vi "Central Commands.vi"(9 "Value":variant, 10 "Commands":T1, 11 "ref in":refnum<k20>) -> (1 "element":T2, 2 "top enqueue?":bool, 3 "ref out":refnum<k20>)   [LabVIEW 2019]
uses:
  RT Controls/Top Process Commands.ctl
  RT Controls/Top Command Events.ctl
  RT Controls/Main Command Events.ctl
  RT Controls/Main Box Config.ctl
  <vilib>/Utility/error.llb/Error Cluster From Error Code.vi
  <vilib>/rvi/errors/niLvFpgaAdjustHostInterfaceError.vi
  <vilib>/rvi/interface/nirviReadWriteControl/nirviReadWriteControl.xnode
  NiFpgaLv.dll
  <vilib>/rvi/interface/Simulation/niFpgaSimulationCallBeginRW.vi
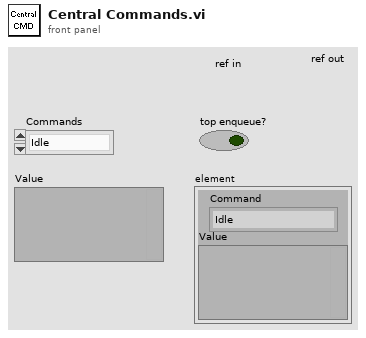
[diagram p1: front panel]
types:
  T1 = typedef "Main Command Events.ctl" = enum16{"Idle", "FullStop", "MainReadConfig", "MainWriteConfig", "OpenUpper", "CloseUpper", "OpenLower", "CloseLower", "SetWatchdogInt", "EnCloudShutDn", "DisCloudShutDn", "SetRainDelay", "EnAutoShutDn", "DisAutoShutDn", "SetRevDelay", "RotToAz", "RotLeft", "RotRight", "RotToHome", "DefineHomePos", "SetHSThres", "SetEncCounts", "SyncClose", "SyncOpen", "SetAZTimLim", "SetAZTol", "AZEncPositive", "AZEncNegative", "RotToCenter"}
  T2 = typedef "Top Process Commands.ctl" = cluster{"Command":T3, "Value":variant}
  T3 = typedef "Top Command Events.ctl" = enum16{"Idle", "FullStop", "ReadConfig", "WriteConfig", "OpenUpper", "CloseUpper", "OpenLower", "CloseLower", "SetWatchdogInt", "EnRainShutDn", "DisRainShutDn", "SetDoorMoveTO", "EnAutoShutDn", "DisAutoShutDn", "SetRevDelay", "SetRainDelay", "SyncClose", "SyncOpen"}
  T4 = typedef "Main Box Config.ctl" = cluster{"WatchdogTim":i32, "DirRevDel":i32, "Coast":dbl, "HSThres":dbl, "EncCounts360":u64, "HomePos":dbl, "EncRefDeg":dbl, "EncRefCounts":u64, "Tol":dbl, "CloudEn":bool, "AutoShutEn":bool, "RainTim":i32, "AZTimeout":i32, "AZEncPol":enum16{"Positive", "Negative"}}
  T5 = cluster{"io.cloud-enable":bool, "io.encoder-negate":bool, "io.encoder-ref":u64, "io.encoder-step":u64, "io.home-pos":fxp<+/-,32,2>, "sm.az-timeout (ms)":u32, "sm.encoder-no-error":u16, "sm.main-pos-hs-thres":fxp<+/-,32,2>, "sm.main-pos-tol":fxp<+/-,32,2>, "sm.cloud-timeout (ms)":u32, "sm.rev-dly (ms)":u32, "io.encoder-center":u64, "sm-main-center-hs-thres":u64, "sm-main-center-tol":u64}
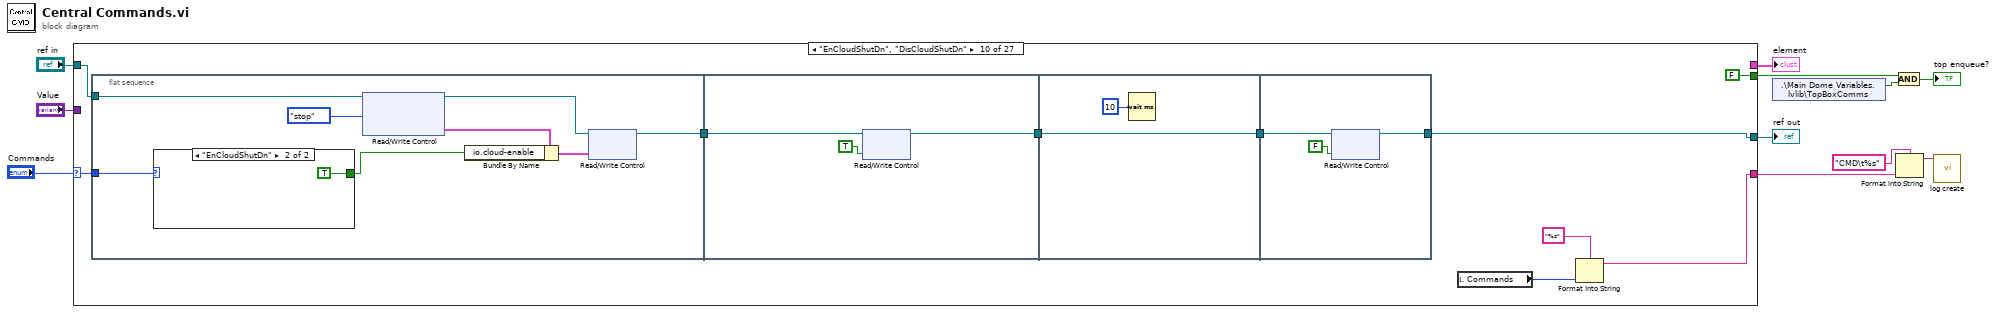
[diagram p0: block diagram]
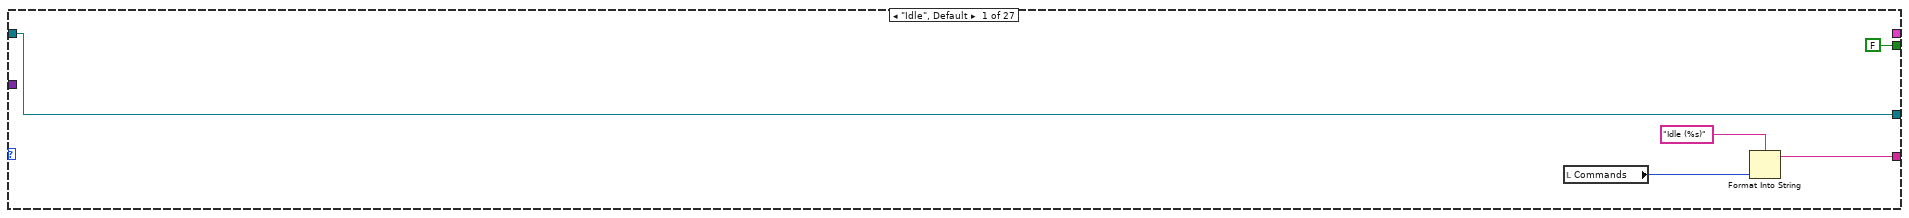
[diagram p2: hidden frame]
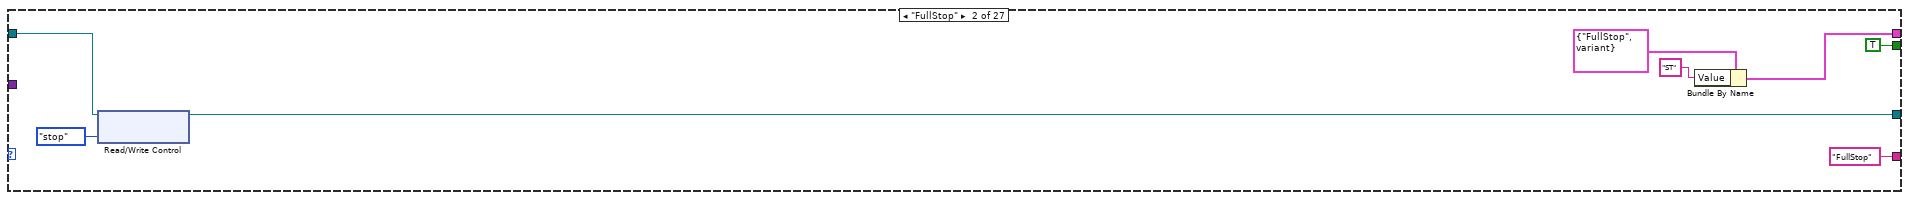
[diagram p3: hidden frame]
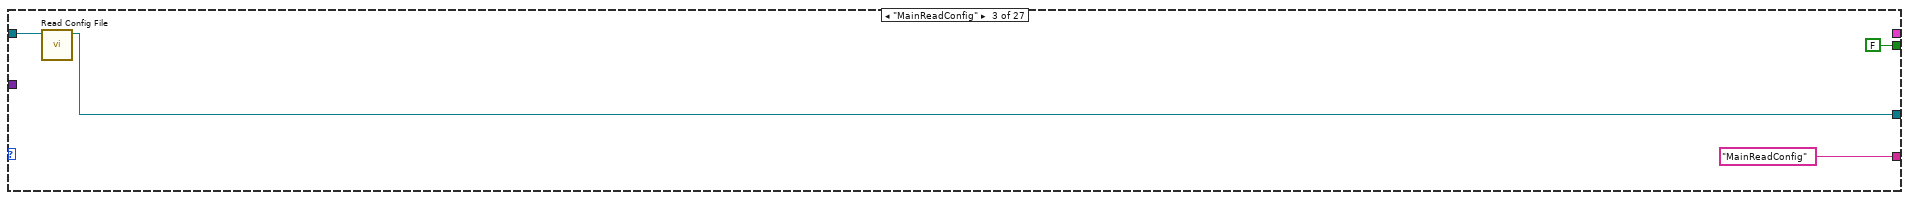
[diagram p4: hidden frame]
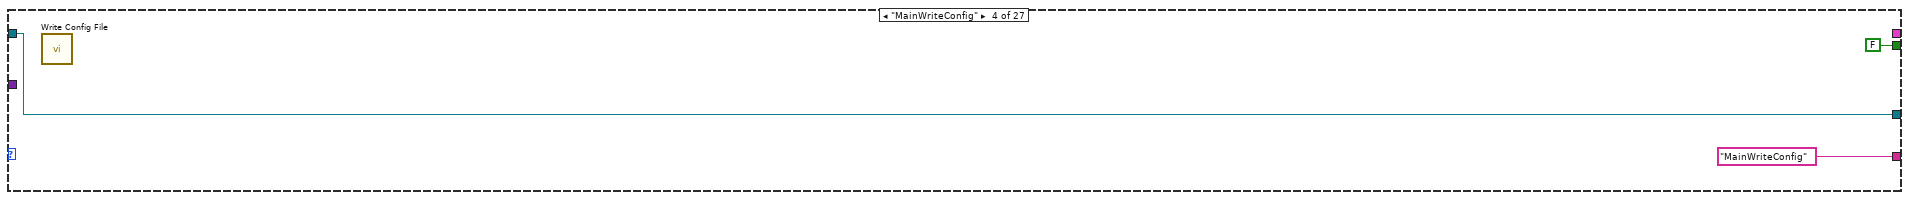
[diagram p5: hidden frame]
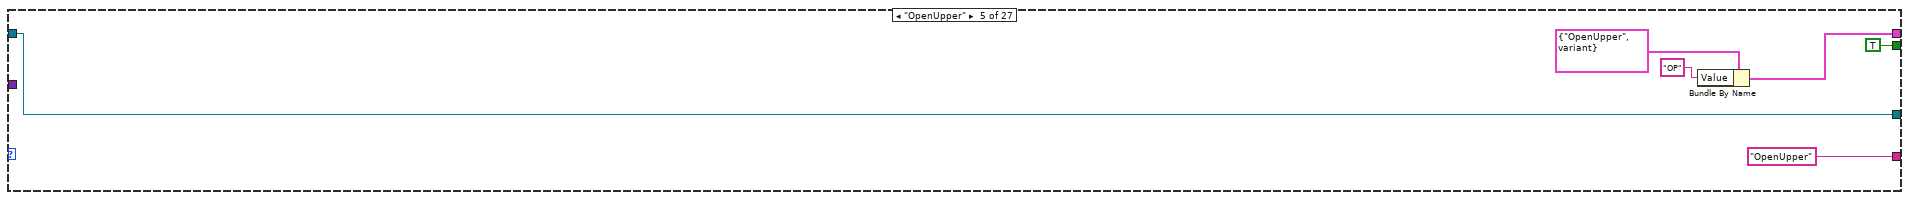
[diagram p6: hidden frame]
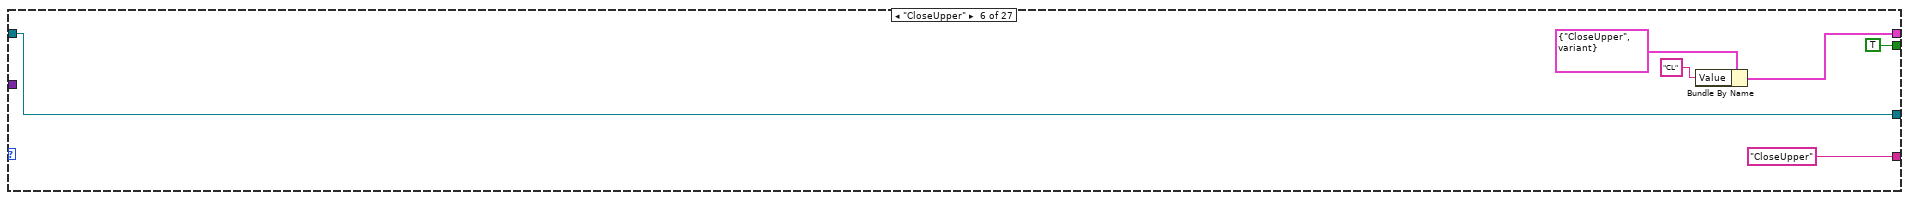
[diagram p7: hidden frame]
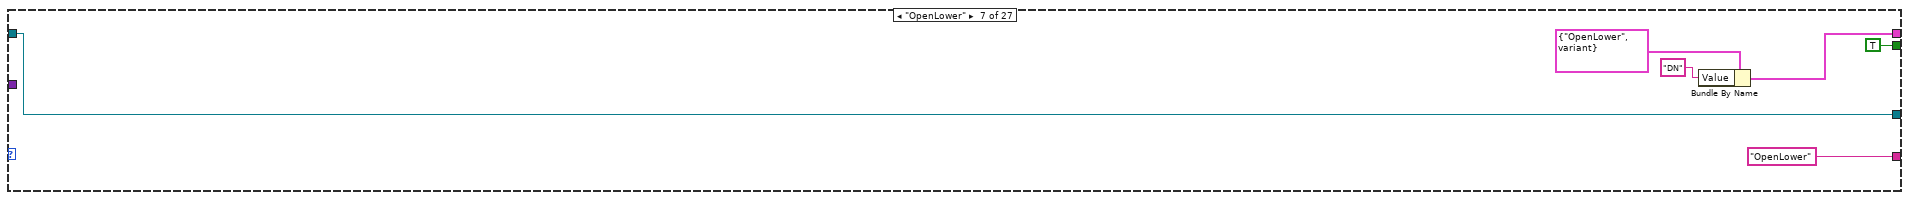
[diagram p8: hidden frame]
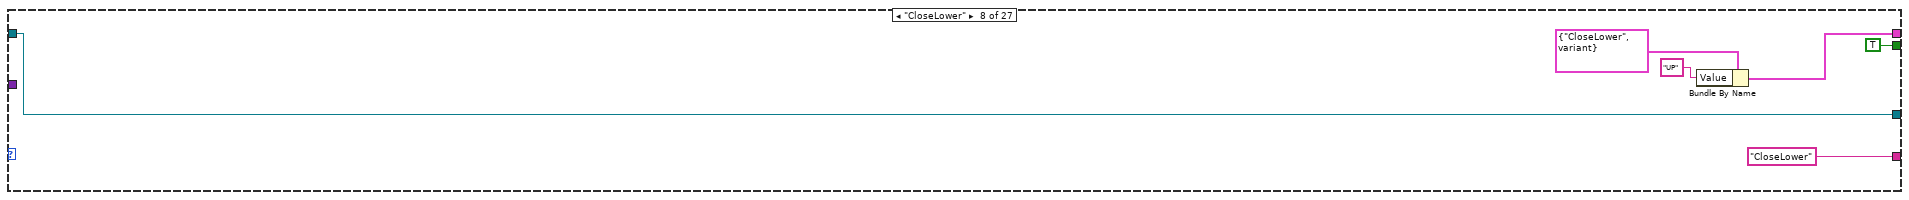
[diagram p9: hidden frame]
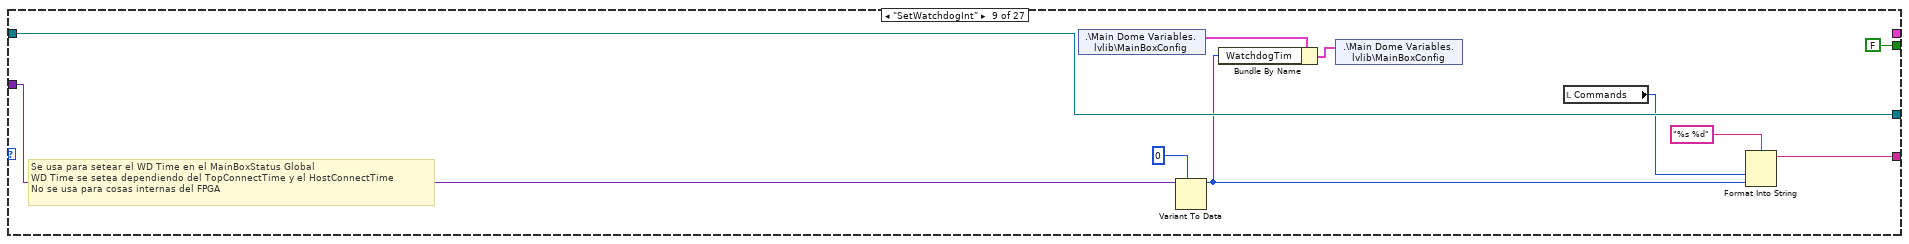
[diagram p10: hidden frame]
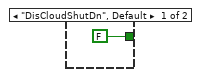
[diagram p11: hidden frame]
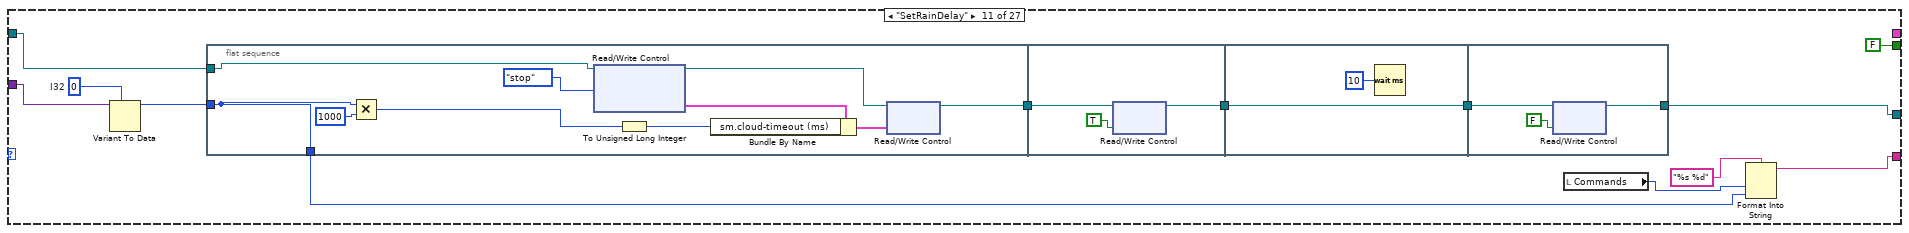
[diagram p12: hidden frame]
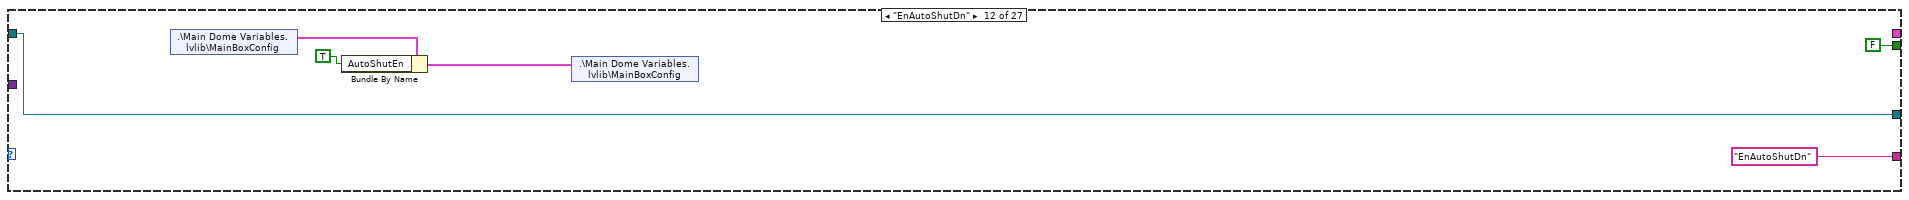
[diagram p13: hidden frame]
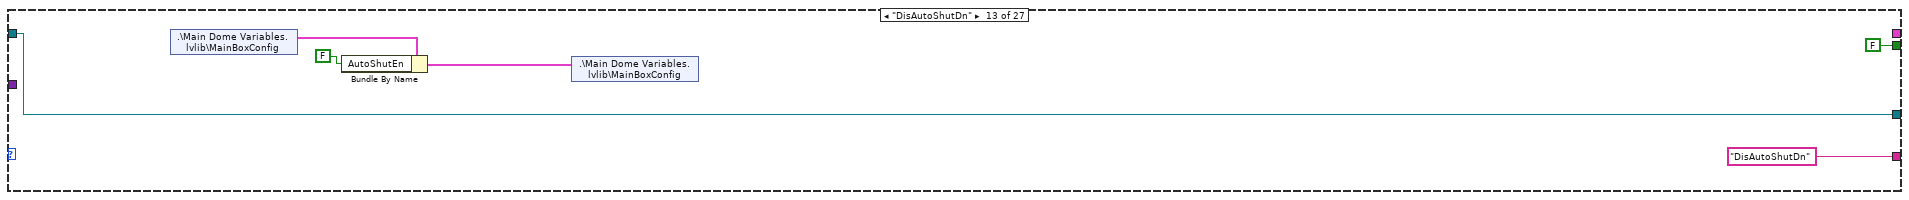
[diagram p14: hidden frame]
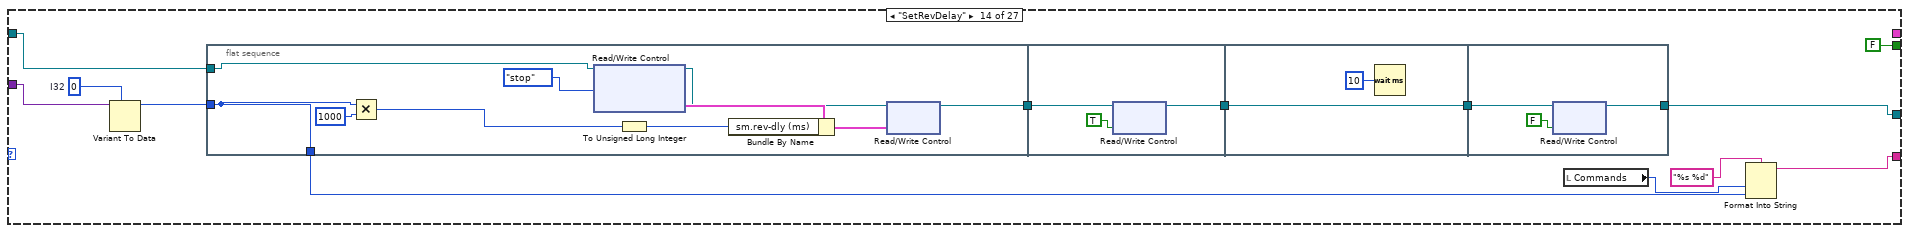
[diagram p15: hidden frame]
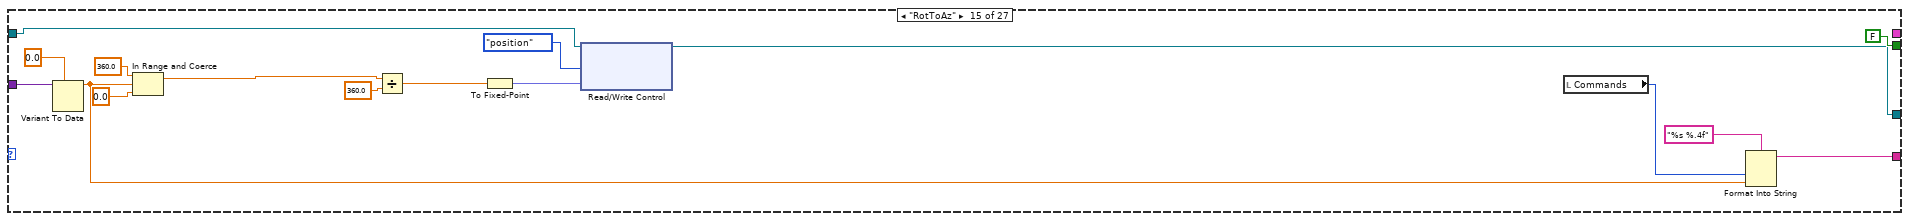
[diagram p16: hidden frame]
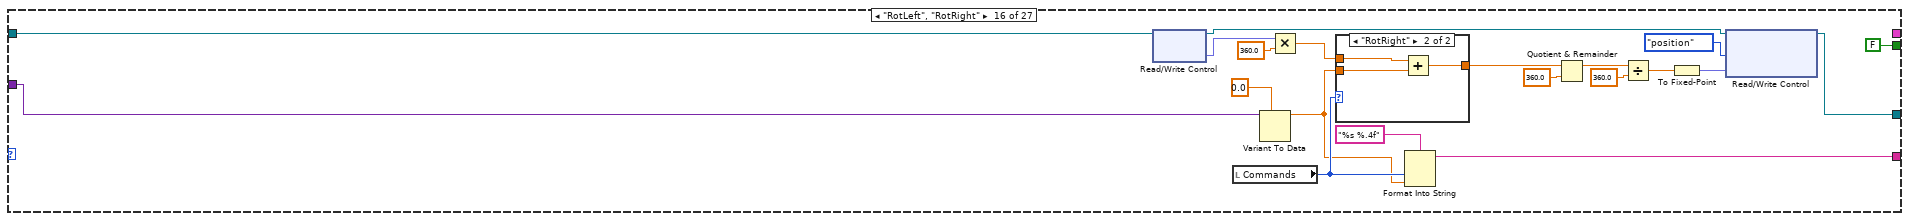
[diagram p17: hidden frame]
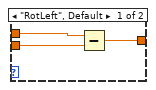
[diagram p18: hidden frame]
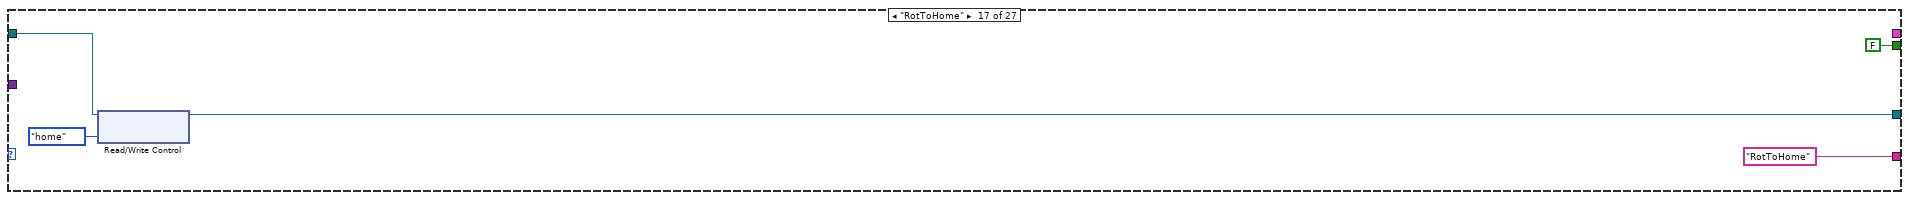
[diagram p19: hidden frame]
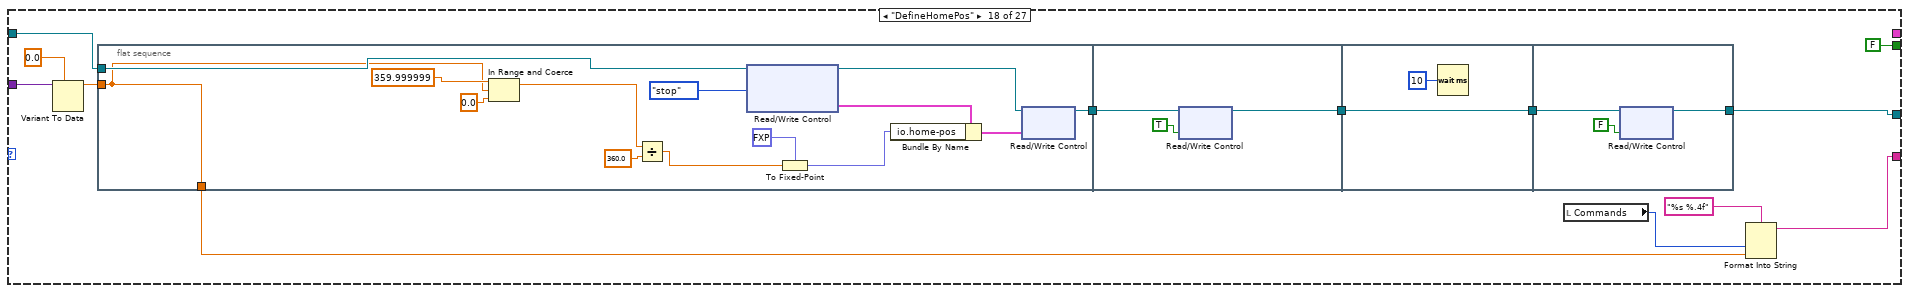
[diagram p20: hidden frame]
diagram:
  n1 = case shown="\"EnCloudShutDn\", \"DisCloudShutDn\"" "Commands" {
    selector: "Commands" -> [_ _ _ _ _ _ _ _ _ w69 _ _ _ _ _ _ _ _ _ _ _ _ _ _ _ _ _]
    tunnel: "Value" -> [_ _ _ _ _ _ _ _ w64 _ w105 _ _ w148 w182 w198 _ w226 w261 w296 _ _ w337 w367 _ _ _]
    tunnel: [FALSE TRUE FALSE FALSE TRUE TRUE TRUE TRUE FALSE FALSE FALSE FALSE FALSE FALSE FALSE FALSE FALSE FALSE FALSE FALSE TRUE TRUE FALSE FALSE FALSE FALSE FALSE] -> w5
    tunnel: [_ w18 _ _ w32 w38 w44 w50 _ _ _ _ _ _ _ _ _ _ _ _ w313 w319 _ _ _ _ _] -> w11
    tunnel: "ref in" -> [w15 w23 w28 w31 w36 w42 w48 w54 w60 w74 w99 w126 w132 w141 w180 w194 w213 w220 w255 w290 w317 w323 w330 w361 w393 w415 w438]
    tunnel: [w15 w22 w27 w31 w36 w42 w48 w54 w60 w70 w98 w126 w132 w143 w173 w197 w212 w219 w254 w289 w317 w323 w329 w360 w392 w414 w437] -> w1
    tunnel: [w12 "FullStop" ("input 1") "MainReadConfig" ("input 1") "MainWriteConfig" ("input 1") "OpenUpper" ("input 1") "CloseUpper" ("input 1") "OpenLower" ("input 1") "CloseLower" ("input 1") w56 w67 w94 "EnAutoShutDn" ("input 1") "DisAutoShutDn" ("input 1") w137 w169 w196 "RotToHome" ("input 1") w215 w250 w285 "SyncClose" ("input 1") "SyncOpen" ("input 1") w325 w356 "AZEncPositive" ("input 1") "AZEncNegative" ("input 1") "RotToCenter" ("input 1")] -> w7
    frame "Idle", Default {
      n2 = local read "Commands"() -> (w13:T1)
      n3 = Format Into String(format string="Idle (%s)", w13) -> (resulting string=w12:string)  [unwired: 2 in, 1 out]
    }
    frame "FullStop" {
      n4 = xnode "Read/Write Control"("FPGA VI Reference In"=w23, "mode request"=enum16{"stop", "home", "position", "center"}."stop") -> ("FPGA VI Reference Out"=w22:refnum<k20>)  [unwired: 1 in, 1 out]
      n5 = Bundle By Name(cluster=T2 {"Command"=enum."FullStop", "Value"=variant} ("element"), "Value"="ST") -> (w18:T2)
    }
    frame "MainReadConfig" {
      n6 = call "Read Config File.vi"("ref in"=w28) -> ("ref out"=w27:refnum<k20>)  [unwired: 10 in]
    }
    frame "MainWriteConfig" {
      n7 = call "Write Config File.vi"() -> ()  [unwired: 12 in]
    }
    frame "OpenUpper" {
      n8 = Bundle By Name(cluster=T2 {"Command"=enum."OpenUpper", "Value"=variant} ("element"), "Value"="OP") -> (w32:T2)
    }
    frame "CloseUpper" {
      n9 = Bundle By Name(cluster=T2 {"Command"=enum."CloseUpper", "Value"=variant} ("element"), "Value"="CL") -> (w38:T2)
    }
    frame "OpenLower" {
      n10 = Bundle By Name(cluster=T2 {"Command"=enum."OpenLower", "Value"=variant} ("element"), "Value"="DN") -> (w44:T2)
    }
    frame "CloseLower" {
      n11 = Bundle By Name(cluster=T2 {"Command"=enum."CloseLower", "Value"=variant} ("element"), "Value"="UP") -> (w50:T2)
    }
    frame "SetWatchdogInt" {
      # "Se usa para setear el WD Time en el MainBoxStatus Global\nWD Time se setea dependiendo del TopConnectTime y el HostConnectTime\nNo se usa para cosas internas del FPGA"
      n12 = shared-variable ".\\Main Dome Variables.lvlib\\MainBoxConfig"() -> (w63:T4)  [unwired: 1 in, 1 out]
      n13 = Variant To Data(type=0 ("number"), Variant=w64) -> (data=w57:i32)  [unwired: 1 in, 1 out]
      n14 = Bundle By Name(cluster=w63, "WatchdogTim"=w57) -> (w62:T4)
      n15 = shared-variable ".\\Main Dome Variables.lvlib\\MainBoxConfig"(w62) -> ()  [unwired: 1 in, 1 out]
      n16 = local read "Commands"() -> (w58:T1)
      n17 = Format Into String(format string="%s %d", w58, w57) -> (resulting string=w56:string)  [unwired: 2 in, 1 out]
    }
    frame "EnCloudShutDn", "DisCloudShutDn" {
      n18 = flat-sequence {
        tunnel: w74 -> [w83]
        tunnel: [w79] -> w73
        tunnel: w69 -> [w78]
        tunnel: w73 -> [w88]
        tunnel: [w86] -> w71
        tunnel: [w89] -> w72
        tunnel: w71 -> [w89]
        tunnel: w72 -> [w92]
        tunnel: [w91] -> w70
        frame #0 {
          n19 = case shown="\"EnCloudShutDn\"" w78 {
            tunnel: [FALSE ("io.cloud-enable") TRUE ("io.cloud-enable")] -> w77
            frame "DisCloudShutDn", Default {
            }
            frame "EnCloudShutDn" {
            }
          }
          n20 = xnode "Read/Write Control"("FPGA VI Reference In"=w83, "mode request"=enum16{"stop", "home", "position", "center"}."stop") -> ("FPGA VI Reference Out"=w81:refnum<k20>, "config"=w82:T5)  [unwired: 1 in, 1 out]
          n21 = Bundle By Name(cluster=w82, "io.cloud-enable"=w77) -> (w80:T5)
          n22 = xnode "Read/Write Control"("FPGA VI Reference In"=w81, "config"=w80) -> ("FPGA VI Reference Out"=w79:refnum<k20>)  [unwired: 1 in, 1 out]
        }
        frame #1 {
          n23 = xnode "Read/Write Control"("FPGA VI Reference In"=w88, "reset"=TRUE) -> ("FPGA VI Reference Out"=w86:refnum<k20>)  [unwired: 1 in, 1 out]
        }
        frame #2 {
          n24 = Wait (ms)(milliseconds to wait=u32 10) -> ()  [unwired: 1 out]
        }
        frame #3 {
          n25 = xnode "Read/Write Control"("FPGA VI Reference In"=w92, "reset"=FALSE) -> ("FPGA VI Reference Out"=w91:refnum<k20>)  [unwired: 1 in, 1 out]
        }
      }
      n26 = local read "Commands"() -> (w66:T1)
      n27 = Format Into String(format string="%s", w66) -> (resulting string=w67:string)  [unwired: 2 in, 1 out]
    }
    frame "SetRainDelay" {
      w106 = 0  # I32
      n28 = Variant To Data(type=w106, Variant=w105) -> (data=w100:i32)  [unwired: 1 in, 1 out]
      n29 = flat-sequence {
        tunnel: w99 -> [w116]
        tunnel: [w112] -> w103
        tunnel: w100 -> [w108]
        tunnel: [w108] -> w95
        tunnel: w103 -> [w119]
        tunnel: [w117] -> w102
        tunnel: [w120] -> w101
        tunnel: w102 -> [w120]
        tunnel: w101 -> [w123]
        tunnel: [w122] -> w98
        frame #0 {
          n30 = Multiply(x=w108, y=1000) -> (x*y=w110:i32)
          n31 = xnode "Read/Write Control"("FPGA VI Reference In"=w116, "mode request"=enum16{"stop", "home", "position", "center"}."stop") -> ("FPGA VI Reference Out"=w114:refnum<k20>, "config"=w115:T5)  [unwired: 1 in, 1 out]
          n32 = To Unsigned Long Integer(number=w110) -> (unsigned 32bit integer=w109:u32)
          n33 = Bundle By Name(cluster=w115, "sm.cloud-timeout (ms)"=w109) -> (w113:T5)
          n34 = xnode "Read/Write Control"("FPGA VI Reference In"=w114, "config"=w113) -> ("FPGA VI Reference Out"=w112:refnum<k20>)  [unwired: 1 in, 1 out]
        }
        frame #1 {
          n35 = xnode "Read/Write Control"("FPGA VI Reference In"=w119, "reset"=TRUE) -> ("FPGA VI Reference Out"=w117:refnum<k20>)  [unwired: 1 in, 1 out]
        }
        frame #2 {
          n36 = Wait (ms)(milliseconds to wait=u32 10) -> ()  [unwired: 1 out]
        }
        frame #3 {
          n37 = xnode "Read/Write Control"("FPGA VI Reference In"=w123, "reset"=FALSE) -> ("FPGA VI Reference Out"=w122:refnum<k20>)  [unwired: 1 in, 1 out]
        }
      }
      n38 = local read "Commands"() -> (w96:T1)
      n39 = Format Into String(format string="%s %d", w96, w95) -> (resulting string=w94:string)  [unwired: 2 in, 1 out]
    }
    frame "EnAutoShutDn" {
      n40 = shared-variable ".\\Main Dome Variables.lvlib\\MainBoxConfig"() -> (w129:T4)  [unwired: 1 in, 1 out]
      n41 = Bundle By Name(cluster=w129, "AutoShutEn"=TRUE ("AllStop")) -> (w128:T4)
      n42 = shared-variable ".\\Main Dome Variables.lvlib\\MainBoxConfig"(w128) -> ()  [unwired: 1 in, 1 out]
    }
    frame "DisAutoShutDn" {
      n43 = shared-variable ".\\Main Dome Variables.lvlib\\MainBoxConfig"() -> (w135:T4)  [unwired: 1 in, 1 out]
      n44 = Bundle By Name(cluster=w135, "AutoShutEn"=FALSE ("AllStop")) -> (w134:T4)
      n45 = shared-variable ".\\Main Dome Variables.lvlib\\MainBoxConfig"(w134) -> ()  [unwired: 1 in, 1 out]
    }
    frame "SetRevDelay" {
      w149 = 0  # I32
      n46 = Variant To Data(type=w149, Variant=w148) -> (data=w142:i32)  [unwired: 1 in, 1 out]
      n47 = flat-sequence {
        tunnel: w141 -> [w159]
        tunnel: [w155] -> w146
        tunnel: w142 -> [w151]
        tunnel: [w151] -> w138
        tunnel: w146 -> [w162]
        tunnel: [w160] -> w145
        tunnel: [w163] -> w144
        tunnel: w145 -> [w163]
        tunnel: w144 -> [w166]
        tunnel: [w165] -> w143
        frame #0 {
          n48 = Multiply(x=w151, y=1000) -> (x*y=w153:i32)
          n49 = xnode "Read/Write Control"("FPGA VI Reference In"=w159, "mode request"=enum16{"stop", "home", "position", "center"}."stop") -> ("FPGA VI Reference Out"=w157:refnum<k20>, "config"=w158:T5)  [unwired: 1 in, 1 out]
          n50 = To Unsigned Long Integer(number=w153) -> (unsigned 32bit integer=w152:u32)
          n51 = Bundle By Name(cluster=w158, "sm.rev-dly (ms)"=w152) -> (w156:T5)
          n52 = xnode "Read/Write Control"("FPGA VI Reference In"=w157, "config"=w156) -> ("FPGA VI Reference Out"=w155:refnum<k20>)  [unwired: 1 in, 1 out]
        }
        frame #1 {
          n53 = xnode "Read/Write Control"("FPGA VI Reference In"=w162, "reset"=TRUE) -> ("FPGA VI Reference Out"=w160:refnum<k20>)  [unwired: 1 in, 1 out]
        }
        frame #2 {
          n54 = Wait (ms)(milliseconds to wait=u32 10) -> ()  [unwired: 1 out]
        }
        frame #3 {
          n55 = xnode "Read/Write Control"("FPGA VI Reference In"=w166, "reset"=FALSE) -> ("FPGA VI Reference Out"=w165:refnum<k20>)  [unwired: 1 in, 1 out]
        }
      }
      n56 = local read "Commands"() -> (w139:T1)
      n57 = Format Into String(format string="%s %d", w139, w138) -> (resulting string=w137:string)  [unwired: 2 in, 1 out]
    }
    frame "RotToAz" {
      n58 = Variant To Data(type=0.0 ("upper limit"), Variant=w182) -> (data=w170:dbl)  [unwired: 1 in, 1 out]
      n59 = In Range and Coerce(upper limit=360.0, x=w170, lower limit=0.0) -> (coerced(x)=w177:dbl)  [unwired: 1 out]
      n60 = Divide(x=w177, y=360.0) -> (x/y=w175:dbl)
      n61 = To Fixed-Point(number=w175) -> (fixed-point=w174:fxp<+/-,32,2>)  [unwired: 1 in]
      n62 = xnode "Read/Write Control"("FPGA VI Reference In"=w180, "mode request"=enum16{"stop", "home", "position", "center"}."position", "az pos req"=w174) -> ("FPGA VI Reference Out"=w173:refnum<k20>)  [unwired: 1 in, 1 out]
      n63 = local read "Commands"() -> (w171:T1)
      n64 = Format Into String(format string="%s %.4f", w171, w170) -> (resulting string=w169:string)  [unwired: 2 in, 1 out]
    }
    frame "RotLeft", "RotRight" {
      n65 = xnode "Read/Write Control"("FPGA VI Reference In"=w194) -> ("FPGA VI Reference Out"=w193:refnum<k20>, "az pos"=w191:fxp<+/-,32,2>)  [unwired: 1 in, 1 out]
      n66 = local read "Commands"() -> (w190:T1)
      n67 = Variant To Data(type=0.0 ("upper limit"), Variant=w198) -> (data=w188:dbl)  [unwired: 1 in, 1 out]
      n68 = Multiply(x=w191, y=360.0 ("upper limit")) -> (x*y=w189:dbl)
      n69 = case shown="\"RotRight\"" w190 {
        tunnel: w189 -> [w205 w209]
        tunnel: w188 -> [w206 w208]
        tunnel: [w204 w207] -> w187
        frame "RotLeft", Default {
          n70 = Subtract(x=w205, y=w206) -> (x-y=w204:dbl)
        }
        frame "RotRight" {
          n71 = Add(x=w209, y=w208) -> (x+y=w207:dbl)
        }
      }
      n72 = Format Into String(format string="%s %.4f", w190, w188) -> (resulting string=w196:string)  [unwired: 2 in, 1 out]
      n73 = Quotient & Remainder(x=w187, y=360.0) -> (x-y*floor(x/y)=w185:dbl)  [unwired: 1 out]
      n74 = Divide(x=w185, y=360.0) -> (x/y=w203:dbl)
      n75 = To Fixed-Point(number=w203) -> (fixed-point=w202:fxp<+/-,32,2>)  [unwired: 1 in]
      n76 = xnode "Read/Write Control"("FPGA VI Reference In"=w193, "mode request"=enum16{"stop", "home", "position", "center"}."position", "az pos req"=w202) -> ("FPGA VI Reference Out"=w197:refnum<k20>)  [unwired: 1 in, 1 out]
    }
    frame "RotToHome" {
      n77 = xnode "Read/Write Control"("FPGA VI Reference In"=w213, "mode request"=enum16{"stop", "home", "position", "center"}."home") -> ("FPGA VI Reference Out"=w212:refnum<k20>)  [unwired: 1 in, 1 out]
    }
    frame "DefineHomePos" {
      n78 = Variant To Data(type=0.0 ("upper limit"), Variant=w226) -> (data=w221:dbl)  [unwired: 1 in, 1 out]
      n79 = flat-sequence {
        tunnel: w220 -> [w241]
        tunnel: [w237] -> w224
        tunnel: w221 -> [w229]
        tunnel: [w229] -> w216
        tunnel: w224 -> [w244]
        tunnel: [w242] -> w223
        tunnel: [w245] -> w222
        tunnel: w223 -> [w245]
        tunnel: w222 -> [w248]
        tunnel: [w247] -> w219
        frame #0 {
          n80 = In Range and Coerce(upper limit=359.999999, x=w229, lower limit=0.0) -> (coerced(x)=w234:dbl)  [unwired: 1 out]
          n81 = Divide(x=w234, y=360.0) -> (x/y=w232:dbl)
          n82 = xnode "Read/Write Control"("FPGA VI Reference In"=w241, "mode request"=enum16{"stop", "home", "position", "center"}."stop") -> ("FPGA VI Reference Out"=w239:refnum<k20>, "config"=w240:T5)  [unwired: 1 in, 1 out]
          n83 = To Fixed-Point(fixed-point type=fxp<+/-,32,2> 0.0 ("az pos req"), number=w232) -> (fixed-point=w230:fxp<+/-,32,2>)
          n84 = Bundle By Name(cluster=w240, "io.home-pos"=w230) -> (w238:T5)
          n85 = xnode "Read/Write Control"("FPGA VI Reference In"=w239, "config"=w238) -> ("FPGA VI Reference Out"=w237:refnum<k20>)  [unwired: 1 in, 1 out]
        }
        frame #1 {
          n86 = xnode "Read/Write Control"("FPGA VI Reference In"=w244, "reset"=TRUE) -> ("FPGA VI Reference Out"=w242:refnum<k20>)  [unwired: 1 in, 1 out]
        }
        frame #2 {
          n87 = Wait (ms)(milliseconds to wait=u32 10) -> ()  [unwired: 1 out]
        }
        frame #3 {
          n88 = xnode "Read/Write Control"("FPGA VI Reference In"=w248, "reset"=FALSE) -> ("FPGA VI Reference Out"=w247:refnum<k20>)  [unwired: 1 in, 1 out]
        }
      }
      n89 = local read "Commands"() -> (w217:T1)
      n90 = Format Into String(format string="%s %.4f", w217, w216) -> (resulting string=w215:string)  [unwired: 2 in, 1 out]
    }
    frame "SetHSThres" {
      n91 = Variant To Data(type=0.0 ("upper limit"), Variant=w261) -> (data=w256:dbl)  [unwired: 1 in, 1 out]
      n92 = flat-sequence {
        tunnel: w255 -> [w276]
        tunnel: [w272] -> w259
        tunnel: w256 -> [w264]
        tunnel: [w264] -> w251
        tunnel: w259 -> [w279]
        tunnel: [w277] -> w258
        tunnel: [w280] -> w257
        tunnel: w258 -> [w280]
        tunnel: w257 -> [w283]
        tunnel: [w282] -> w254
        frame #0 {
          n93 = In Range and Coerce(upper limit=359.999999, x=w264, lower limit=0.0) -> (coerced(x)=w269:dbl)  [unwired: 1 out]
          n94 = Divide(x=w269, y=360.0) -> (x/y=w267:dbl)
          n95 = xnode "Read/Write Control"("FPGA VI Reference In"=w276, "mode request"=enum16{"stop", "home", "position", "center"}."stop") -> ("FPGA VI Reference Out"=w274:refnum<k20>, "config"=w275:T5)  [unwired: 1 in, 1 out]
          n96 = To Fixed-Point(fixed-point type=fxp<+/-,32,2> 0.0 ("az pos req"), number=w267) -> (fixed-point=w265:fxp<+/-,32,2>)
          n97 = Bundle By Name(cluster=w275, "sm.main-pos-hs-thres"=w265) -> (w273:T5)
          n98 = xnode "Read/Write Control"("FPGA VI Reference In"=w274, "config"=w273) -> ("FPGA VI Reference Out"=w272:refnum<k20>)  [unwired: 1 in, 1 out]
        }
        frame #1 {
          n99 = xnode "Read/Write Control"("FPGA VI Reference In"=w279, "reset"=TRUE) -> ("FPGA VI Reference Out"=w277:refnum<k20>)  [unwired: 1 in, 1 out]
        }
        frame #2 {
          n100 = Wait (ms)(milliseconds to wait=u32 10) -> ()  [unwired: 1 out]
        }
        frame #3 {
          n101 = xnode "Read/Write Control"("FPGA VI Reference In"=w283, "reset"=FALSE) -> ("FPGA VI Reference Out"=w282:refnum<k20>)  [unwired: 1 in, 1 out]
        }
      }
      n102 = local read "Commands"() -> (w252:T1)
      n103 = Format Into String(format string="%s %.4f", w252, w251) -> (resulting string=w250:string)  [unwired: 2 in, 1 out]
    }
    frame "SetEncCounts" {
      n104 = Variant To Data(type=u64 0 ("upper limit"), Variant=w296) -> (data=w291:u64)  [unwired: 1 in, 1 out]
      n105 = flat-sequence {
        tunnel: w290 -> [w304]
        tunnel: [w300] -> w294
        tunnel: w291 -> [w299]
        tunnel: [w299] -> w287
        tunnel: w294 -> [w307]
        tunnel: [w305] -> w293
        tunnel: [w308] -> w292
        tunnel: w293 -> [w308]
        tunnel: w292 -> [w311]
        tunnel: [w310] -> w289
        frame #0 {
          n106 = xnode "Read/Write Control"("FPGA VI Reference In"=w304, "mode request"=enum16{"stop", "home", "position", "center"}."stop") -> ("FPGA VI Reference Out"=w302:refnum<k20>, "config"=w303:T5)  [unwired: 1 in, 1 out]
          n107 = Bundle By Name(cluster=w303, "io.encoder-step"=w299) -> (w301:T5)
          n108 = xnode "Read/Write Control"("FPGA VI Reference In"=w302, "config"=w301) -> ("FPGA VI Reference Out"=w300:refnum<k20>)  [unwired: 1 in, 1 out]
        }
        frame #1 {
          n109 = xnode "Read/Write Control"("FPGA VI Reference In"=w307, "reset"=TRUE) -> ("FPGA VI Reference Out"=w305:refnum<k20>)  [unwired: 1 in, 1 out]
        }
        frame #2 {
          n110 = Wait (ms)(milliseconds to wait=u32 10) -> ()  [unwired: 1 out]
        }
        frame #3 {
          n111 = xnode "Read/Write Control"("FPGA VI Reference In"=w311, "reset"=FALSE) -> ("FPGA VI Reference Out"=w310:refnum<k20>)  [unwired: 1 in, 1 out]
        }
      }
      n112 = local read "Commands"() -> (w286:T1)
      n113 = Format Into String(format string="%s %d", w286, w287) -> (resulting string=w285:string)  [unwired: 2 in, 1 out]
    }
    frame "SyncClose" {
      n114 = Bundle By Name(cluster=T2 {"Command"=enum."SyncClose", "Value"=variant} ("element"), "Value"="SC") -> (w313:T2)
    }
    frame "SyncOpen" {
      n115 = Bundle By Name(cluster=T2 {"Command"=enum."SyncOpen", "Value"=variant} ("element"), "Value"="SO") -> (w319:T2)
    }
    frame "SetAZTimLim" {
      n116 = Variant To Data(type=0 ("upper limit"), Variant=w337) -> (data=w331:i32)  [unwired: 1 in, 1 out]
      n117 = flat-sequence {
        tunnel: w330 -> [w347]
        tunnel: [w343] -> w334
        tunnel: w331 -> [w339]
        tunnel: [w339] -> w327
        tunnel: w334 -> [w350]
        tunnel: [w348] -> w333
        tunnel: [w351] -> w332
        tunnel: w333 -> [w351]
        tunnel: w332 -> [w354]
        tunnel: [w353] -> w329
        frame #0 {
          n118 = Multiply(x=w339, y=1000) -> (x*y=w341:i32)
          n119 = xnode "Read/Write Control"("FPGA VI Reference In"=w347, "mode request"=enum16{"stop", "home", "position", "center"}."stop") -> ("FPGA VI Reference Out"=w345:refnum<k20>, "config"=w346:T5)  [unwired: 1 in, 1 out]
          n120 = To Unsigned Long Integer(number=w341) -> (unsigned 32bit integer=w340:u32)
          n121 = Bundle By Name(cluster=w346, "sm.az-timeout (ms)"=w340) -> (w344:T5)
          n122 = xnode "Read/Write Control"("FPGA VI Reference In"=w345, "config"=w344) -> ("FPGA VI Reference Out"=w343:refnum<k20>)  [unwired: 1 in, 1 out]
        }
        frame #1 {
          n123 = xnode "Read/Write Control"("FPGA VI Reference In"=w350, "reset"=TRUE) -> ("FPGA VI Reference Out"=w348:refnum<k20>)  [unwired: 1 in, 1 out]
        }
        frame #2 {
          n124 = Wait (ms)(milliseconds to wait=u32 10) -> ()  [unwired: 1 out]
        }
        frame #3 {
          n125 = xnode "Read/Write Control"("FPGA VI Reference In"=w354, "reset"=FALSE) -> ("FPGA VI Reference Out"=w353:refnum<k20>)  [unwired: 1 in, 1 out]
        }
      }
      n126 = local read "Commands"() -> (w326:T1)
      n127 = Format Into String(format string="%s %d", w326, w327) -> (resulting string=w325:string)  [unwired: 2 in, 1 out]
    }
    frame "SetAZTol" {
      n128 = Variant To Data(type=0.0 ("upper limit"), Variant=w367) -> (data=w362:dbl)  [unwired: 1 in, 1 out]
      n129 = flat-sequence {
        tunnel: w361 -> [w382]
        tunnel: [w378] -> w365
        tunnel: w362 -> [w370]
        tunnel: [w370] -> w358
        tunnel: w365 -> [w385]
        tunnel: [w383] -> w364
        tunnel: [w386] -> w363
        tunnel: w364 -> [w386]
        tunnel: w363 -> [w389]
        tunnel: [w388] -> w360
        frame #0 {
          n130 = In Range and Coerce(upper limit=359.999999, x=w370, lower limit=0.0) -> (coerced(x)=w375:dbl)  [unwired: 1 out]
          n131 = Divide(x=w375, y=360.0) -> (x/y=w373:dbl)
          n132 = xnode "Read/Write Control"("FPGA VI Reference In"=w382, "mode request"=enum16{"stop", "home", "position", "center"}."stop") -> ("FPGA VI Reference Out"=w380:refnum<k20>, "config"=w381:T5)  [unwired: 1 in, 1 out]
          n133 = To Fixed-Point(fixed-point type=fxp<+/-,32,2> 0.0 ("az pos req"), number=w373) -> (fixed-point=w371:fxp<+/-,32,2>)
          n134 = Bundle By Name(cluster=w381, "sm.main-pos-tol"=w371) -> (w379:T5)
          n135 = xnode "Read/Write Control"("FPGA VI Reference In"=w380, "config"=w379) -> ("FPGA VI Reference Out"=w378:refnum<k20>)  [unwired: 1 in, 1 out]
        }
        frame #1 {
          n136 = xnode "Read/Write Control"("FPGA VI Reference In"=w385, "reset"=TRUE) -> ("FPGA VI Reference Out"=w383:refnum<k20>)  [unwired: 1 in, 1 out]
        }
        frame #2 {
          n137 = Wait (ms)(milliseconds to wait=u32 10) -> ()  [unwired: 1 out]
        }
        frame #3 {
          n138 = xnode "Read/Write Control"("FPGA VI Reference In"=w389, "reset"=FALSE) -> ("FPGA VI Reference Out"=w388:refnum<k20>)  [unwired: 1 in, 1 out]
        }
      }
      n139 = local read "Commands"() -> (w357:T1)
      n140 = Format Into String(format string="%s %.4f", w357, w358) -> (resulting string=w356:string)  [unwired: 2 in, 1 out]
    }
    frame "AZEncPositive" {
      n141 = flat-sequence {
        tunnel: w393 -> [w404]
        tunnel: [w400] -> w396
        tunnel: w396 -> [w407]
        tunnel: [w405] -> w395
        tunnel: [w408] -> w394
        tunnel: w395 -> [w408]
        tunnel: w394 -> [w411]
        tunnel: [w410] -> w392
        frame #0 {
          n142 = xnode "Read/Write Control"("FPGA VI Reference In"=w404, "mode request"=enum16{"stop", "home", "position", "center"}."stop") -> ("FPGA VI Reference Out"=w402:refnum<k20>, "config"=w403:T5)  [unwired: 1 in, 1 out]
          n143 = Bundle By Name(cluster=w403, "io.encoder-negate"=FALSE) -> (w401:T5)
          n144 = xnode "Read/Write Control"("FPGA VI Reference In"=w402, "config"=w401) -> ("FPGA VI Reference Out"=w400:refnum<k20>)  [unwired: 1 in, 1 out]
        }
        frame #1 {
          n145 = xnode "Read/Write Control"("FPGA VI Reference In"=w407, "reset"=TRUE) -> ("FPGA VI Reference Out"=w405:refnum<k20>)  [unwired: 1 in, 1 out]
        }
        frame #2 {
          n146 = Wait (ms)(milliseconds to wait=u32 10) -> ()  [unwired: 1 out]
        }
        frame #3 {
          n147 = xnode "Read/Write Control"("FPGA VI Reference In"=w411, "reset"=FALSE) -> ("FPGA VI Reference Out"=w410:refnum<k20>)  [unwired: 1 in, 1 out]
        }
      }
    }
    frame "AZEncNegative" {
      n148 = flat-sequence {
        tunnel: w415 -> [w426]
        tunnel: [w422] -> w418
        tunnel: w418 -> [w429]
        tunnel: [w427] -> w417
        tunnel: [w430] -> w416
        tunnel: w417 -> [w430]
        tunnel: w416 -> [w433]
        tunnel: [w432] -> w414
        frame #0 {
          n149 = xnode "Read/Write Control"("FPGA VI Reference In"=w426, "mode request"=enum16{"stop", "home", "position", "center"}."stop") -> ("FPGA VI Reference Out"=w424:refnum<k20>, "config"=w425:T5)  [unwired: 1 in, 1 out]
          n150 = Bundle By Name(cluster=w425, "io.encoder-negate"=TRUE) -> (w423:T5)
          n151 = xnode "Read/Write Control"("FPGA VI Reference In"=w424, "config"=w423) -> ("FPGA VI Reference Out"=w422:refnum<k20>)  [unwired: 1 in, 1 out]
        }
        frame #1 {
          n152 = xnode "Read/Write Control"("FPGA VI Reference In"=w429, "reset"=TRUE) -> ("FPGA VI Reference Out"=w427:refnum<k20>)  [unwired: 1 in, 1 out]
        }
        frame #2 {
          n153 = Wait (ms)(milliseconds to wait=u32 10) -> ()  [unwired: 1 out]
        }
        frame #3 {
          n154 = xnode "Read/Write Control"("FPGA VI Reference In"=w433, "reset"=FALSE) -> ("FPGA VI Reference Out"=w432:refnum<k20>)  [unwired: 1 in, 1 out]
        }
      }
    }
    frame "RotToCenter" {
      n155 = xnode "Read/Write Control"("FPGA VI Reference In"=w438, "mode request"=enum16{"stop", "home", "position", "center"}."center") -> ("FPGA VI Reference Out"=w437:refnum<k20>)  [unwired: 1 in, 1 out]
    }
  }
  "element" <- w11
  "ref out" <- w1
  n156 = shared-variable ".\\Main Dome Variables.lvlib\\TopBoxComms"() -> (w4:bool)  [unwired: 1 in, 1 out]
  n157 = And(x=w5, y=w4) -> (x .and. y?=→"top enqueue?":bool)
  n158 = Format Into String(format string="CMD\t%s", w7) -> (resulting string=w6:string)  [unwired: 2 in, 1 out]
  n159 = call "log create.vi"("message"=w6) -> ()  [unwired: 11 in]
